vi "UI.vi"() -> ()   [LabVIEW 2016, in "流量计集成.lvlib" / "LS-H600流量计.lvlib"]
uses:
  SL1500-3G/Ctl/modbus output data.ctl
  <vilib>/Utility/miscctls.llb/LVPointTypeDef.ctl
  <vilib>/Plasmionique/MB Master/MB_Master_Serial/MB_Master_Serial.lvclass
  D:/Program Files (x86)/National Instruments/LabVIEW 2016/vi.lib/Plasmionique/MB Master/MB_Master/MB_Master.lvclass
  <vilib>/Plasmionique/MB Master/MB Master.lvlib
  SL1500-3G/SL1500-3G.lvlib
panel:
  in  "运行模式":enum16{"维护模式", "常规模式"}(ring)=enum."常规模式"
  out "Modbus Data Output":T1
  in  "串口打开":bool
  in  "serial port":refnum<visa-resource-name> caption="串口"
  in  "baud rate":u32(ring)=19200 caption="波特率" items=["1200"=1200, "2400"=2400, "4800"=4800, "9600"=9600, "19200"=19200, "38400"=38400, "115200"=115200]
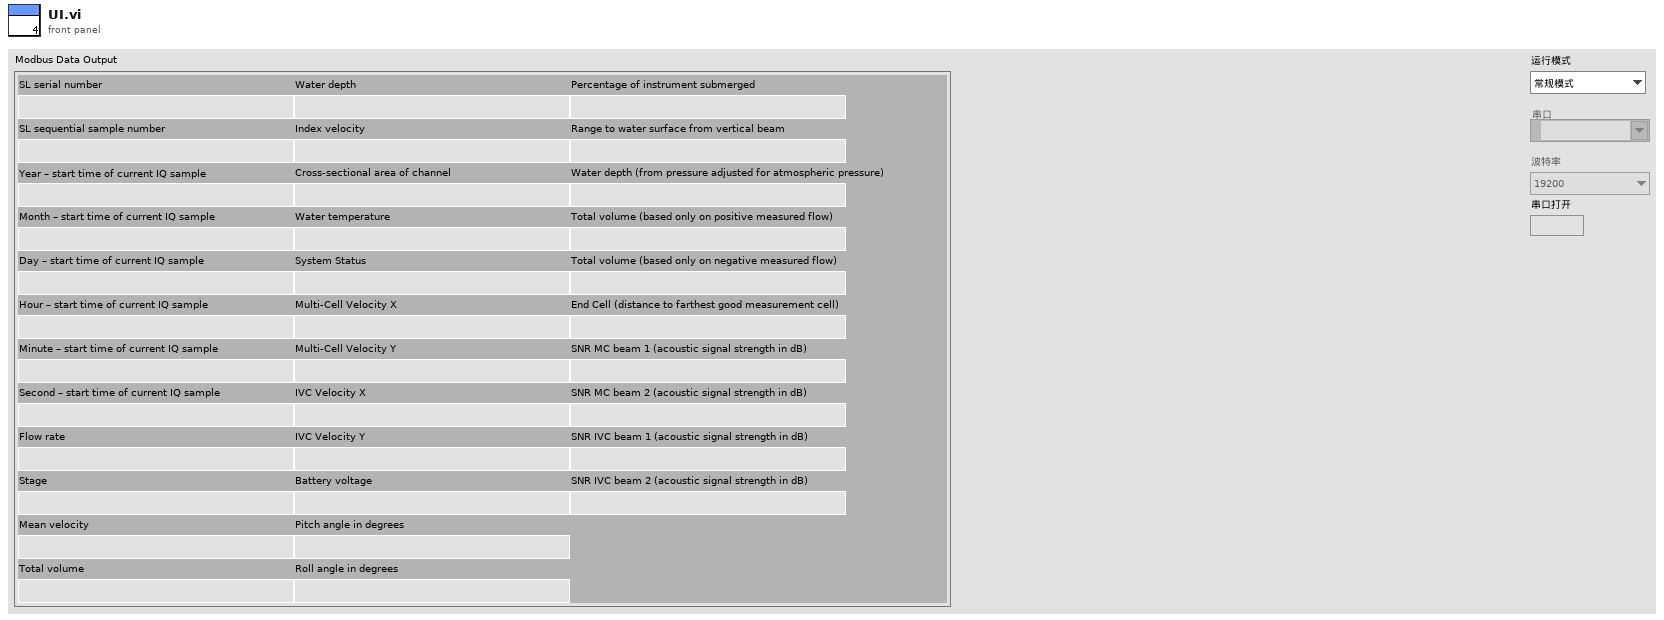
[diagram p1: front panel]
types:
  T1 = typedef "流量计集成.lvlib/SL1500-3G.lvlib/modbus output data.ctl" = cluster{"SL serial number":dbl, "SL sequential sample number":dbl, "Year – start time of current IQ sample":dbl, "Month – start time of current IQ sample":dbl, "Day – start time of current IQ sample":dbl, "Hour – start time of current IQ sample":dbl, "Minute – start time of current IQ sample":dbl, "Second – start time of current IQ sample":dbl, "Flow rate":dbl, "Stage":dbl, "Mean velocity":dbl, "Total volume":dbl, "Water depth":dbl, "Index velocity":dbl, "Cross-sectional area of channel":dbl, "Water temperature":dbl, "System Status":dbl, "Multi-Cell Velocity X":dbl, "Multi-Cell Velocity Y":dbl, "IVC Velocity X":dbl, "IVC Velocity Y":dbl, "Battery voltage":dbl, "Pitch angle in degrees":dbl, "Roll angle in degrees":dbl, "Percentage of instrument submerged":dbl, "Range to water surface from vertical beam":dbl, "Water depth (from pressure adjusted for atmospheric pressure)":dbl, "Total volume (based only on positive measured flow)":dbl, "Total volume (based only on negative measured flow)":dbl, "End Cell (distance to farthest good measurement cell)":dbl, "SNR MC beam 1 (acoustic signal strength in dB)":dbl, "SNR MC beam 2 (acoustic signal strength in dB)":dbl, "SNR IVC beam 1 (acoustic signal strength in dB)":dbl, "SNR IVC beam 2 (acoustic signal strength in dB)":dbl}
  T2 = typedef "LVPointTypeDef.ctl" = cluster{"Horizontal":i16, "Vertical":i16}
  T3 = typedef "LVDateTimeRec.ctl" = cluster{"秒数的小数部分":dbl, "秒":i32, "分":i32, "时":i32, "日":i32, "月":i32, "年":i32, "天数（周）":i32, "天数（年）":i32, "DST":i32}
  T4 = typedef "SL1500-3G.lvlib/modbus output data.ctl" = cluster{"SL serial number":dbl, "SL sequential sample number":dbl, "Year – start time of current IQ sample":dbl, "Month – start time of current IQ sample":dbl, "Day – start time of current IQ sample":dbl, "Hour – start time of current IQ sample":dbl, "Minute – start time of current IQ sample":dbl, "Second – start time of current IQ sample":dbl, "Flow rate":dbl, "Stage":dbl, "Mean velocity":dbl, "Total volume":dbl, "Water depth":dbl, "Index velocity":dbl, "Cross-sectional area of channel":dbl, "Water temperature":dbl, "System Status":dbl, "Multi-Cell Velocity X":dbl, "Multi-Cell Velocity Y":dbl, "IVC Velocity X":dbl, "IVC Velocity Y":dbl, "Battery voltage":dbl, "Pitch angle in degrees":dbl, "Roll angle in degrees":dbl, "Percentage of instrument submerged":dbl, "Range to water surface from vertical beam":dbl, "Water depth (from pressure adjusted for atmospheric pressure)":dbl, "Total volume (based only on positive measured flow)":dbl, "Total volume (based only on negative measured flow)":dbl, "End Cell (distance to farthest good measurement cell)":dbl, "SNR MC beam 1 (acoustic signal strength in dB)":dbl, "SNR MC beam 2 (acoustic signal strength in dB)":dbl, "SNR IVC beam 1 (acoustic signal strength in dB)":dbl, "SNR IVC beam 2 (acoustic signal strength in dB)":dbl}
  T5 = cluster{"baud rate (bps)":u32, "stop bits":u16, "parity":u16, "flow control":u16, "timeout":u32, "retries":i32}
  T6 = enum8{"Enabled", "Disabled", "Disabled and Grayed Out"}
  T7 = cluster{"[0]":sgl, "[1]":sgl, "[2]":sgl, "[3]":sgl, "[4]":sgl, "[5]":sgl, "[6]":sgl, "[7]":sgl, "[8]":sgl, "[9]":sgl, "[10]":sgl, "[11]":sgl, "[12]":sgl, "[13]":sgl, "[14]":sgl, "[15]":sgl, "[16]":sgl, "[17]":sgl, "[18]":sgl, "[19]":sgl, "[20]":sgl, "[21]":sgl, "[22]":sgl, "[23]":sgl, "[24]":sgl, "[25]":sgl, "[26]":sgl, "[27]":sgl, "[28]":sgl, "[29]":sgl, "[30]":sgl, "[31]":sgl, "[32]":sgl, "[33]":sgl}
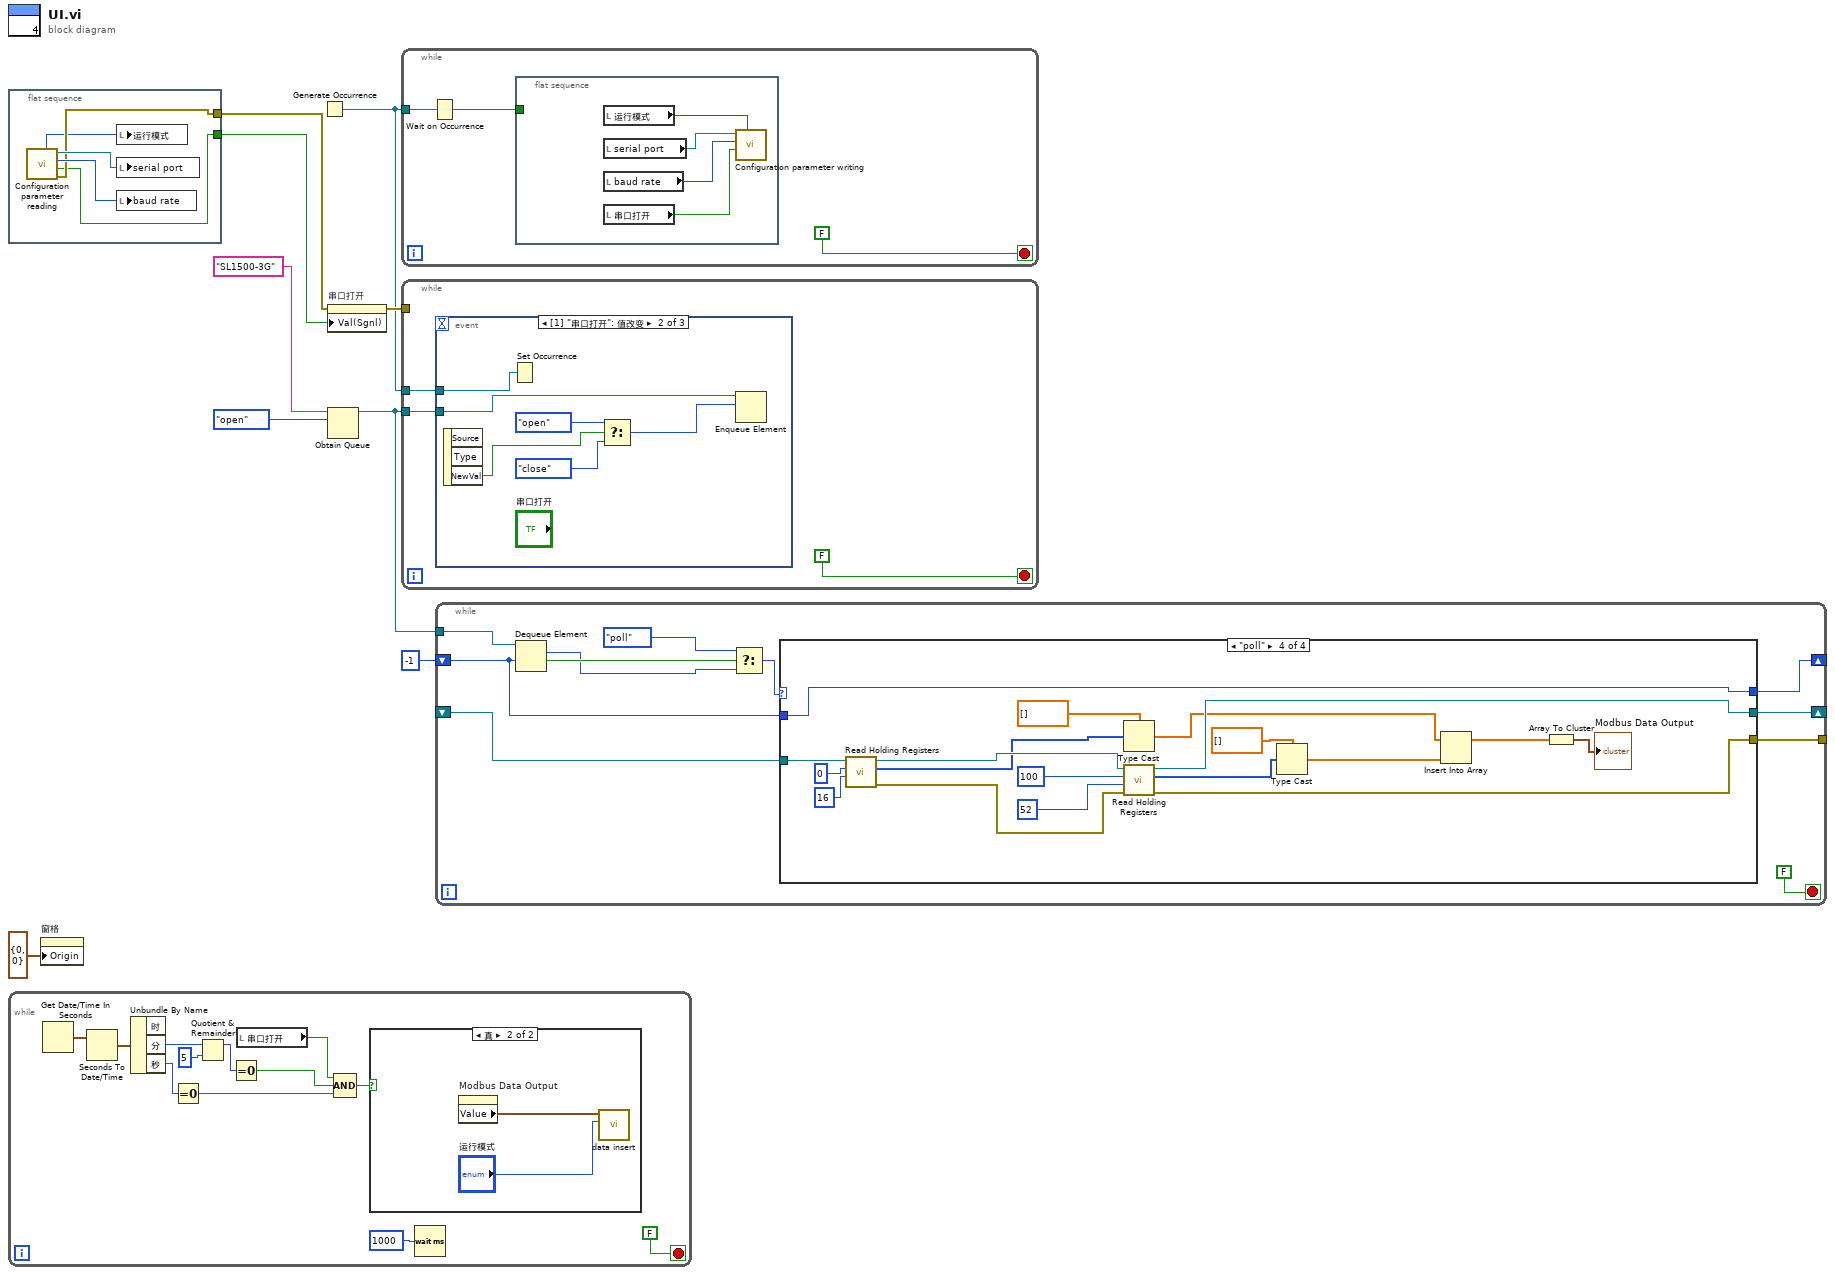
[diagram p0: block diagram]
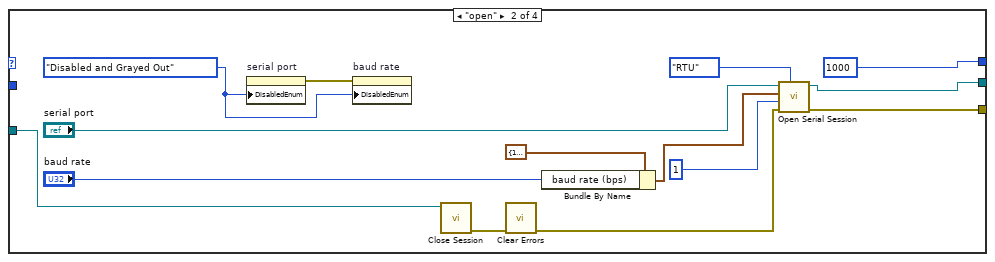
[diagram p4: hidden frame]
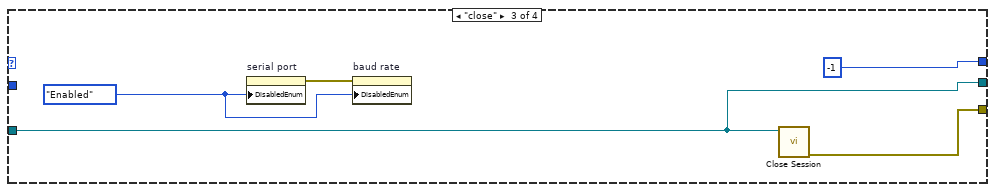
[diagram p5: hidden frame]
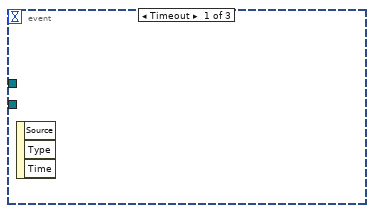
[diagram p6: hidden frame]
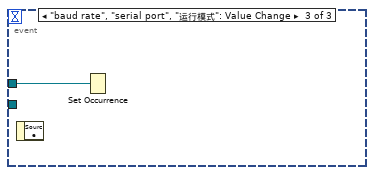
[diagram p7: hidden frame]
diagram:
  n1 = flat-sequence {
    tunnel: [w12] -> w3
    tunnel: [w11] -> w1
    frame #0 {
      n2 = call "Configuration parameter reading.vi"() -> ("error out"=w12:errorcluster, "串口打开"=w11:bool, "baud rate (9600)"=w13:u32, "VISA resource name"=w14:refnum<visa-resource-name>, "运行模式"=w10:enum16{"维护模式", "常规模式"})  [unwired: 7 in]
      n3 = local write "运行模式"(w10) -> ()
      n4 = local write "serial port"(w14) -> ()
      n5 = local write "baud rate"(w13) -> ()
    }
  }
  n6 = while {
    stop <- FALSE stop-if-true
    n7 = Get Date/Time In Seconds() -> (seconds since 1Jan1904=w25:timestamp)
    n8 = Seconds To Date/Time(time stamp (now)=w25) -> (date time rec=w24:T3)  [unwired: 1 in]
    n9 = Unbundle By Name(w24) -> ("分"=w18:i32, "秒"=w22:i32)  [unwired: 1 out]
    n10 = Equal To 0?(x=w22) -> (x = 0?=w19:bool)
    n11 = Quotient & Remainder(x=w18, y=5) -> (x-y*floor(x/y)=w21:i32)  [unwired: 1 out]
    n12 = Equal To 0?(x=w21) -> (x = 0?=w20:bool)
    n13 = local read "串口打开"() -> (w17:bool)
    n14 = Compound Arithmetic op=AND ("复合运算")(w17, w20, w19) -> (w15:bool)
    n15 = case shown="真" w15 {
      frame False {
      }
      frame True {
        n16 = property on="Modbus Data Output" class="Clust (严格)"() -> ("Value"=w28:T4)  [unwired: 2 in, 2 out]
        n17 = call "data insert.vi"("运行模式"="运行模式", "modbus-data"=w28) -> ()  [unwired: 9 in, 1 out]
      }
    }
    n18 = Wait (ms)(milliseconds to wait=u32 1000 ("等待时间（毫秒）")) -> ()  [unwired: 1 out]
  }
  n19 = property on="窗格" class="Pane"("Origin"=T2 {"Horizontal"=0, "Vertical"=0} ("原点")) -> ()  [unwired: 2 in, 2 out]
  n20 = Generate Occurrence() -> (w2:refnum<k4>)
  n21 = property on="串口打开" class="Bool (严格)"(error in=w3, "Val(Sgnl)"=w1) -> (error out=w6:errorcluster)  [unwired: 1 in, 1 out]
  n22 = Obtain Queue(name (unnamed)="SL1500-3G" ("名称（未命名）"), element data type=enum16{"open", "close", "poll"}."open" ("枚举")) -> (queue out=w5:refnum<queue>)  [unwired: 3 in, 2 out]
  n23 = while {
    tunnel: w2 -> [w30]
    stop <- FALSE stop-if-true
    n24 = Wait on Occurrence(2:w30) -> (0:w29:bool)  [unwired: 2 in]
    n25 = flat-sequence {
      tunnel: w29 -> [_]
      frame #0 {
        n26 = local read "运行模式"() -> (w34:enum16{"维护模式", "常规模式"})
        n27 = local read "serial port"() -> (w33:refnum<visa-resource-name>)
        n28 = local read "baud rate"() -> (w32:u32)
        n29 = local read "串口打开"() -> (w35:bool)
        n30 = call "Configuration parameter writing.vi"("运行模式"=w34, "串口打开"=w35, "baud rate (9600)"=w32, "VISA resource name"=w33) -> ()  [unwired: 7 in, 1 out]
      }
    }
  }
  n31 = while {
    tunnel: w6 -> [_]
    tunnel: w5 -> [w37]
    tunnel: w2 -> [w36]
    stop <- FALSE stop-if-true
    n32 = event shown="[1] \"串口打开\": 值改变" {
      selector: _ -> [_ _ _]
      dyn-events: _ -> [_ _ _]
      timeout: _ -> [_ _ _]
      tunnel: w37 -> [_ w43 _]
      tunnel: w36 -> [_ w39 w45]
      event Timeout {
        n33 = event-data() -> ()  [unwired: 1 in, 3 out]
      }
      event "串口打开": Value Change {
        n34 = event-data() -> ("NewVal"=w44:bool)  [unwired: 1 in, 2 out]
        n35 = Set Occurrence(w39) -> ()
        n36 = Select(t=enum16{"open", "close", "poll"}."open" ("元素"), s=w44, f=enum16{"open", "close", "poll"}."close" ("元素")) -> (s? t:f=w40:enum16{"open", "close", "poll"})
        n37 = Enqueue Element(queue=w43, element=w40) -> ()  [unwired: 2 in, 3 out]
      }
      event "baud rate", "serial port", "运行模式": Value Change {
        n38 = event-data() -> ()  [unwired: 1 in, 1 out]
        n39 = Set Occurrence(w45) -> ()
      }
    }
  }
  n40 = while {
    tunnel: w5 -> [w56]
    shift-right: [w55] -> _
    shift-left: _ -> [w54]
    tunnel: [w53] -> _
    shift-right: [w51] -> _
    shift-left: -1 -> [w50]
    stop <- FALSE stop-if-true
    n41 = Dequeue Element(queue=w56, timeout in ms (-1)=w50) -> (element=w48:enum16{"open", "close", "poll"}, timed out?=w49:bool)  [unwired: 1 in, 2 out]
    n42 = Select(t=enum16{"open", "close", "poll"}."poll", s=w49, f=w48) -> (s? t:f=w47:enum16{"open", "close", "poll"})
    n43 = case shown="\"poll\"" w47 {
      tunnel: [w58 w72 w76 w88] -> w55
      tunnel: w54 -> [w58 w71 w76 w95]
      tunnel: [_ w64 w77 w87] -> w53
      tunnel: [w57 1000 -1 w78] -> w51
      tunnel: w50 -> [w57 _ _ w78]
      frame Default {
      }
      frame "open" {
        w61 = T6."Disabled and Grayed Out" ("禁用")
        n44 = property on="serial port" class="VISAName"("DisabledEnum"=w61) -> (error out=w60:errorcluster)  [unwired: 2 in, 1 out]
        n45 = property on="baud rate" class="Ring (严格)"(error in=w60, "DisabledEnum"=w61) -> ()  [unwired: 1 in, 2 out]
        n46 = call-dynamic "Close Session.vi"("MB_Serial session"=w71) -> ("error out"=w63:errorcluster)  [unwired: 10 in]
        n47 = call <vilib>:"Clear Errors.vi"("error in (no error)"=w63) -> ("error out"=w62:errorcluster)  [unwired: 5 in, 1 out]
        n48 = Bundle By Name(cluster=T5 {"baud rate (bps)"=19200, "stop bits"=10, "parity"=0, "flow control"=0, "timeout"=1000, "retries"=1} ("Serial Config"), "baud rate (bps)"="baud rate") -> (w67:T5)
        n49 = call <vilib>:"Open Serial Session.vi"("Mode (RTU)"=enum16{"RTU", "ASCII"}."RTU", "Error in"=w62, "Slave ID"=u8 1, "Serial Config"=w67, "VISA Resource"="serial port") -> ("Error out"=w64:errorcluster, "MB_Serial session"=w72:refnum<class "MB_Master_Serial.lvclass">)  [unwired: 5 in]
      }
      frame "close" {
        w75 = T6."Enabled" ("禁用")
        n50 = property on="serial port" class="VISAName"("DisabledEnum"=w75) -> (error out=w74:errorcluster)  [unwired: 2 in, 1 out]
        n51 = property on="baud rate" class="Ring (严格)"(error in=w74, "DisabledEnum"=w75) -> ()  [unwired: 1 in, 2 out]
        n52 = call-dynamic "Close Session.vi"("MB_Serial session"=w76) -> ("error out"=w77:errorcluster)  [unwired: 10 in]
      }
      frame "poll" {
        n53 = call <vilib>:"Read Holding Registers.vi"("quantity"=u16 16, "starting address"=u16 0, "MB session in"=w95) -> ("error out"=w91:errorcluster, "Registers"=w86:u16[], "MB session out"=w92:refnum<class "MB_Master_Serial.lvclass">)  [unwired: 6 in]
        n54 = Type Cast(type=sgl[] [], x=w86) -> (*(type *) &x=w82:sgl[])
        n55 = call <vilib>:"Read Holding Registers.vi"("error in (no error)"=w91, "quantity"=u16 52, "starting address"=u16 100, "MB session in"=w92) -> ("error out"=w87:errorcluster, "Registers"=w83:u16[], "MB session out"=w88:refnum<class "MB_Master_Serial.lvclass">)  [unwired: 5 in]
        n56 = Type Cast(type=sgl[] [], x=w83) -> (*(type *) &x=w81:sgl[])
        n57 = Insert Into Array(array=w82, new element=w81) -> (w80:sgl[])  [unwired: 1 in]
        n58 = Array To Cluster(array=w80) -> (cluster=→"Modbus Data Output":T7)
      }
    }
  }
